vi "Get Type.vi"(8 "error in (no error)":errorcluster, 11 "Battery Stack in":refnum<class "Battery Stack.lvclass">) -> (0 "error out":errorcluster, 2 "Item Type":T1, 3 "Battery Stack out":refnum<class "Battery Stack.lvclass">)   [LabVIEW 2020, in "Battery Stack.lvclass"]
uses:
  Battery Stack.lvclass
  Item/Item Type.ctl
  Item/Item.lvclass
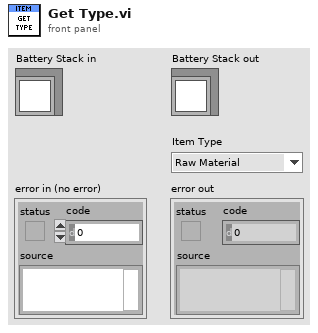
[diagram p1: front panel]
types:
  T1 = typedef "Item.lvclass/Item Type.ctl" = enum16{"Raw Material", "Component", "Module", "Product"}
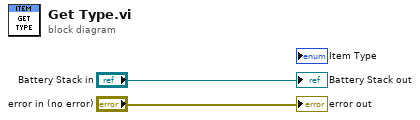
[diagram p0: block diagram]
diagram:
  "error out" <- "error in (no error)"
  "Battery Stack out" <- "Battery Stack in"
